vi "Global_CMD_ACT_Data In.vi"() -> ()   [LabVIEW 2023, in "Extend_ACT.lvlib"]
uses:
  Extend_ACT.lvlib
  Cluster_CMD_ACT_Data.ctl
  2024 Ripon Swerve Source/Shared Code/TypeDefs/ENUM_Extend_CMD_Mode Select.ctl
panel:
  in  "CMD_ACT_Extend_Data":T1
  # "The Names of the Data items in the Global Variable MUST describe who the Single Writer is\nFor Command Globals the Commander(CMD) represents Teleop or Autonomous or other command loop.\nThe naming convention for a Command Actuator Global is:   \n\nCMD_ACT_SubSystem_Data Name\n\nExample:\nCMD_ACT_Drive_Data\nCMD_ACT_Hopper_Eject Ball"
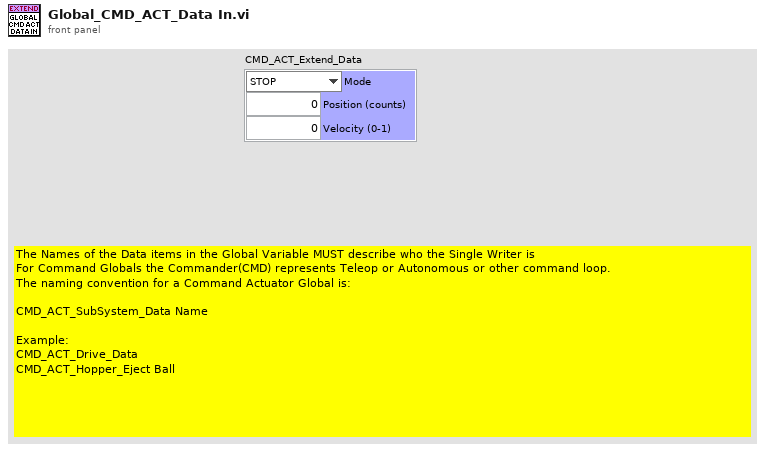
[diagram p1: front panel]
types:
  T1 = typedef "Extend_ACT.lvlib/Cluster_CMD_ACT_Data.ctl" = cluster{"Mode":T2, "Position (counts)":i32, "Velocity (0-1)":dbl}
  T2 = typedef "ENUM_Extend_CMD_Mode Select.ctl" = enum16{"STOP", "Position", "Velocity", "Force Home"}
diagram:
